vi "Add(U16).vi"(1 "Enable(T)":bool=TRUE, 2 "In":u16, 4 "n":u16=1) -> (6 "Out":u16=1)   [LabVIEW 2013]
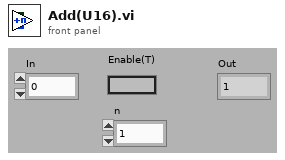
[diagram p1: front panel]
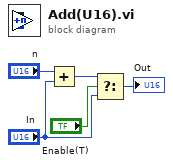
[diagram p0: block diagram]
diagram:
  n1 = Add(x="n", y="In") -> (x+y=w1:u16)
  n2 = Select(t=w1, s="Enable(T)", f="In") -> (s? t:f=→"Out":u16)
